vi "CNN.vi"() -> ()   [LabVIEW 2018]
panel:
  out "Image Classes":i32[](array[numeric])
  out "Character Images":picture[](array[picture])
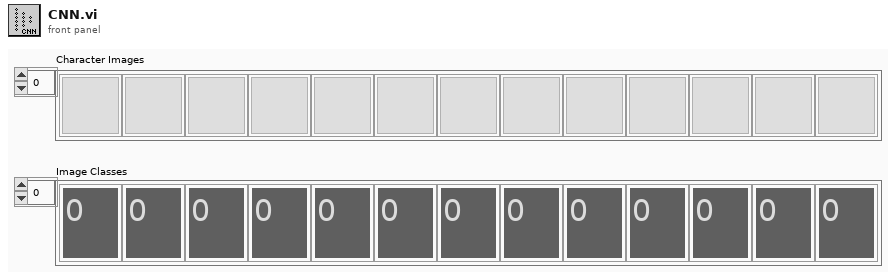
[diagram p1: front panel]
types:
  T1 = cluster{"Stride":i32, "Offset - x":i32, "Offset - y":i32, "Round Up":bool}
  T2 = cluster{"Stride":i32, "Offset - x":i32, "Offset - y":i32, "Size Mode":enum16{"Round Up", "Round Down", "Same"}}
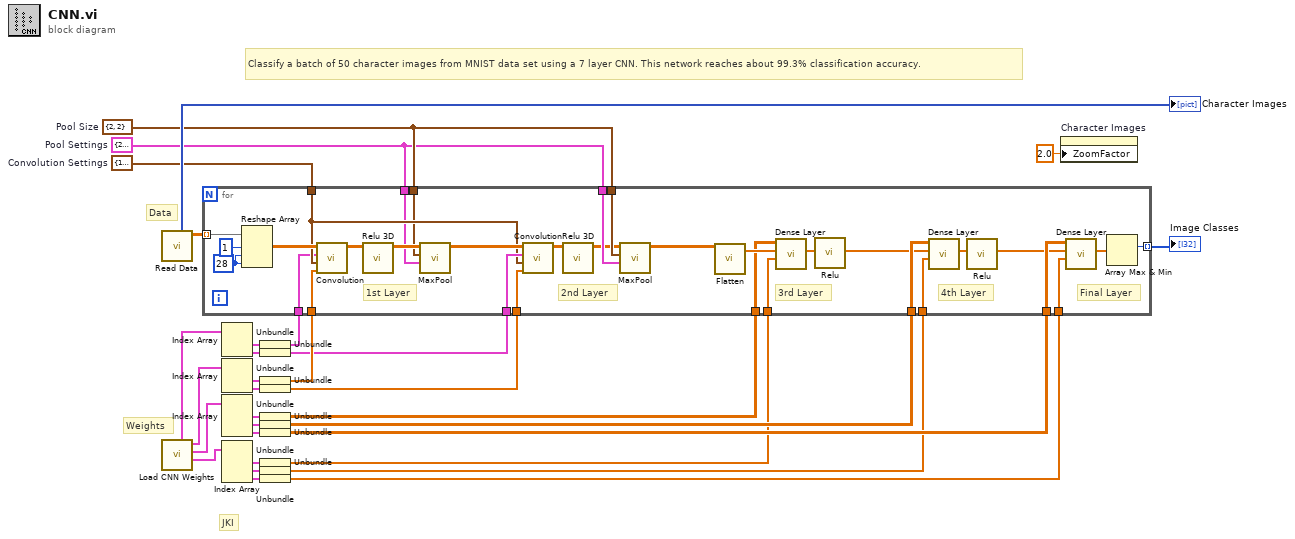
[diagram p0: block diagram]
diagram:
  w12 = T1 {"Stride"=2, "Offset - x"=0, "Offset - y"=0, "Round Up"=TRUE}  # Pool Settings
  w13 = cluster{"X Size":i32, "Y Size":i32} {"X Size"=2, "Y Size"=2}  # Pool Size
  w20 = T2 {"Stride"=1, "Offset - x"=2, "Offset - y"=2, "Size Mode"=enum."Same"}  # Convolution Settings
  # "JKI"
  # "Weights"
  # "Data"
  # "Classify a batch of 50 character images from MNIST data set using a 7 layer CNN. This network reaches about 99.3% classification accuracy."
  n1 = call "Read Data.vi"() -> ("Normalized Data"=w25:dbl[][], "Character Images"=→"Character Images":picture[])  [unwired: 9 in, 1 out]
  n2 = call "Load CNN Weights.vi"() -> ("Dense Layer - Biases"=w26:cluster{"Data out":dbl[]}[], "Dense Layer - Weights"=w27:cluster{dbl[][]}[], "Convolutional Layer - Biases"=w28:cluster{dbl[]}[], "Convolutional Layer - Kernals"=w29:cluster{cluster{dbl[][][]}[]}[])  [unwired: 7 in, 1 out]
  n3 = Index Array(array=w29) -> (element #1=w11:cluster{cluster{dbl[][][]}[]}, element #2=w19:cluster{cluster{dbl[][][]}[]})  [unwired: 2 in]
  n4 = Index Array(array=w28) -> (element #1=w24:cluster{dbl[]}, element #2=w18:cluster{dbl[]})  [unwired: 2 in]
  n5 = Index Array(array=w27) -> (element #1=w23:cluster{dbl[][]}, element #2=w17:cluster{dbl[][]}, element #3=w15:cluster{dbl[][]})  [unwired: 3 in]
  n6 = Index Array(array=w26) -> (element #1=w22:cluster{"Data out":dbl[]}, element #2=w16:cluster{"Data out":dbl[]}, element #3=w14:cluster{"Data out":dbl[]})  [unwired: 3 in]
  n7 = Unbundle(w11) -> (w10:cluster{dbl[][][]}[])
  n8 = Unbundle(w19) -> (w8:cluster{dbl[][][]}[])
  n9 = Unbundle(w24) -> (w9:dbl[])
  n10 = Unbundle(w18) -> (w7:dbl[])
  n11 = Unbundle(w23) -> (w6:dbl[][])
  n12 = Unbundle(w17) -> (w5:dbl[][])
  n13 = Unbundle(w15) -> (w4:dbl[][])
  n14 = Unbundle(w22) -> ("Data out"=w3:dbl[])
  n15 = Unbundle(w16) -> ("Data out"=w2:dbl[])
  n16 = Unbundle(w14) -> ("Data out"=w1:dbl[])
  n17 = for {
    tunnel: w8 -> [w56]
    tunnel: w9 -> [w55]
    tunnel: w7 -> [w54]
    tunnel: w6 -> [w53]
    tunnel: w5 -> [w52]
    tunnel: w3 -> [w51]
    tunnel: w2 -> [w50]
    tunnel: w25 -> [w49] mode=indexing
    tunnel: [w47] -> w21 mode=indexing
    tunnel: w20 -> [w46]
    tunnel: w4 -> [w45]
    tunnel: w1 -> [w44]
    tunnel: w13 -> [w42]
    tunnel: w12 -> [w41]
    tunnel: w13 -> [w40]
    tunnel: w12 -> [w39]
    tunnel: w10 -> [w32]
    w62 = 28 ("dimension size")
    # "Final Layer"
    # "4th Layer"
    # "3rd Layer"
    # "2nd Layer"
    # "1st Layer"
    n18 = Reshape Array(w49, 1 ("dimension size"), w62, w62) -> (w58:dbl[][][])
    n19 = call "Convolution.vi"("Bias"=w55, "Convolution Settings"=w46, "Kernals"=w32, "Data In"=w58) -> ("Data Out"=w57:dbl[][][])  [unwired: 7 in]
    n20 = call "Relu 3D.vi"("Data In"=w57) -> ("Data out"=w48:dbl[][][])  [unwired: 10 in]
    n21 = call "MaxPool.vi"("Convolution Settings"=w41, "Pool Size"=w42, "Data In"=w48) -> ("Data Out"=w59:dbl[][][])  [unwired: 8 in]
    n22 = call "Convolution.vi"("Bias"=w54, "Convolution Settings"=w46, "Kernals"=w56, "Data In"=w59) -> ("Data Out"=w38:dbl[][][])  [unwired: 7 in]
    n23 = call "Relu 3D.vi"("Data In"=w38) -> ("Data out"=w37:dbl[][][])  [unwired: 10 in]
    n24 = call "MaxPool.vi"("Convolution Settings"=w39, "Pool Size"=w40, "Data In"=w37) -> ("Data Out"=w61:dbl[][][])  [unwired: 8 in]
    n25 = call "Flatten.vi"("Data Out in"=w61) -> ("Data Out out"=w60:dbl[])  [unwired: 10 in]
    n26 = call "Dense Layer.vi"("Bias (1xb)"=w51, "Data X (1xa)"=w60, "Weights (axb)"=w53) -> ("Output Y (1xb)"=w34:dbl[])  [unwired: 8 in]
    n27 = call "Relu.vi"("Data In"=w34) -> ("Data out"=w33:dbl[])  [unwired: 10 in]
    n28 = call "Dense Layer.vi"("Bias (1xb)"=w50, "Data X (1xa)"=w33, "Weights (axb)"=w52) -> ("Output Y (1xb)"=w36:dbl[])  [unwired: 8 in]
    n29 = call "Relu.vi"("Data In"=w36) -> ("Data out"=w35:dbl[])  [unwired: 10 in]
    n30 = call "Dense Layer.vi"("Bias (1xb)"=w44, "Data X (1xa)"=w35, "Weights (axb)"=w45) -> ("Output Y (1xb)"=w43:dbl[])  [unwired: 8 in]
    n31 = Array Max & Min(array=w43) -> (max index (indices)=w47:i32)  [unwired: 3 out]
  }
  "Image Classes" <- w21
  n32 = property on="Character Images" class="Pict"("ZoomFactor"=sgl 2.0 ("Zoom Factor")) -> ()  [unwired: 2 in, 2 out]
